vi "Get Experiement All Devices.vi"(9 "Experiment name":string, 10 "RingText.Text 2":string, 11 "RingText.Text":string) -> (3 "> Filtered Device List>":string[](array[string]))   [LabVIEW 2020]
uses:
  Shared/MySQL/Preset Query Enum.ctl
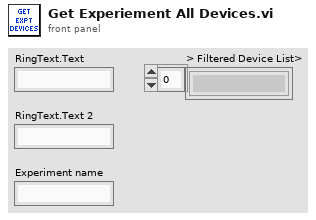
[diagram p1: front panel]
types:
  T1 = typedef "Preset Query Enum.ctl" = enum16{"Get Locations", "Get all IPs and MACs", "Get classes", "Get expt variables to set at scanstart for particular device", "Get expt devices and variables with start values", "Get expt devices and variables (with data to get)", "Get expt devices with data to get", "Get Expt devices and GUIs", "Get all devices basic properties", "Get Virtual Devices Core Info", "Get Expt names", "Get experiment basic properties", "Get experiment alarm variables", "Get MC Ports", "Get device network comm port", "Get devicetype lvclass path", "Get basic device properties", "Get Init Order", "Get all setable variables of a device", "Get device variable aliases", "Get force values of all settable variables", "Get all variables of a devicetype", "Get all variables of a device", "Get plotter details", "Get Saved Scans", "Get Scan Info", "GetGeneralGUIs", "Get expt for plotter", "Get plotter IDs from expt", "Get all devices", "Get all Virtual Devices", "Get all aliases", "Get variable and device info for Virtual Device", "GetItemLocatorIP", "Get IPs for GUIs", "Get DeviceType from Device", "GetLocalPortRange", "GetDevicePresetVariables", "Get Device Configuration", "GetAllPresetNames", "GetAllConfigurationNames", "GetPresetDeviceNames"}
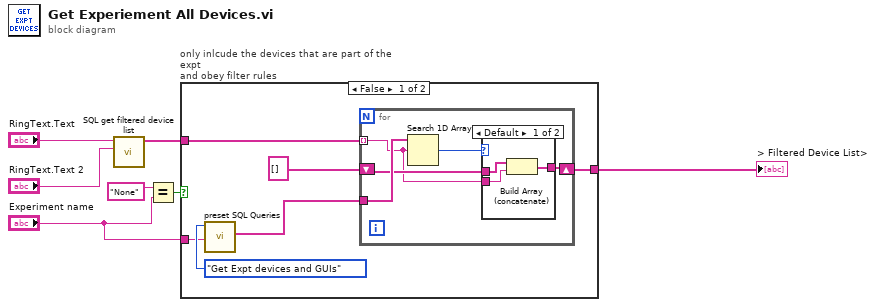
[diagram p0: block diagram]
diagram:
  n1 = call "SQL get filtered device list.vi"("class"="RingText.Text 2", "location"="RingText.Text") -> ("filtered device list"=w3:string[])  [unwired: 8 in, 1 out]
  n2 = Equal?(x="None", y="Experiment name") -> (x = y?=w5:bool)
  n3 = case "only inlcude the devices that are part of the expt\nand obey filter rules" shown="False" w5 {
    tunnel: w3 -> [w13 w23]
    tunnel: [w12 w23] -> w7
    tunnel: "Experiment name" -> [w9 _]
    frame False {
      n4 = call "preset SQL Queries.vi"("Expt name / MCIP/ Variable/Preset Name"=w9, "Preset Query"=Preset_Query_Enum."Get Expt devices and GUIs") -> ("1st column 1st data"=w8:string[])  [unwired: 7 in, 2 out]
      n5 = for {
        tunnel: w13 -> [w14] mode=indexing
        tunnel: w8 -> [w18]
        shift-right: [w16] -> w12
        shift-left: string[] [] -> [w15]
        n6 = Search 1D Array(1D array=w18, element=w14) -> (index of element=w17:i32)  [unwired: 1 in]
        n7 = case shown="Default" w17 {
          tunnel: [w21 w22] -> w16
          tunnel: w15 -> [w19 w22]
          tunnel: w14 -> [w20 _]
          frame Default {
            n8 = Build Array (concatenate)(w19, w20) -> (w21:string[])
          }
          frame -1 {
          }
        }
      }
    }
    frame True {
    }
  }
  "> Filtered Device List>" <- w7
